vi "enigma.vi"() -> ()   [LabVIEW 2023]
panel:
  in  "Pistoketaulu":string[][](array[combo])
  in  "Kiekko 3":string(combo)
  in  "Kiekko 2":string(combo)
  in  "Kiekko 1":string(combo)
  in  "Kiekot":dbl[](array[numeric]) min=1.0 max=3.0 step=1.0
  in  "III":string(combo)
  in  "II":string(combo)
  in  "I":string(combo)
  out "Teksti ulos":string
  in  "Teksti sisään":string
  # "Aloitus"
  # "Kiekkojen asetukset"
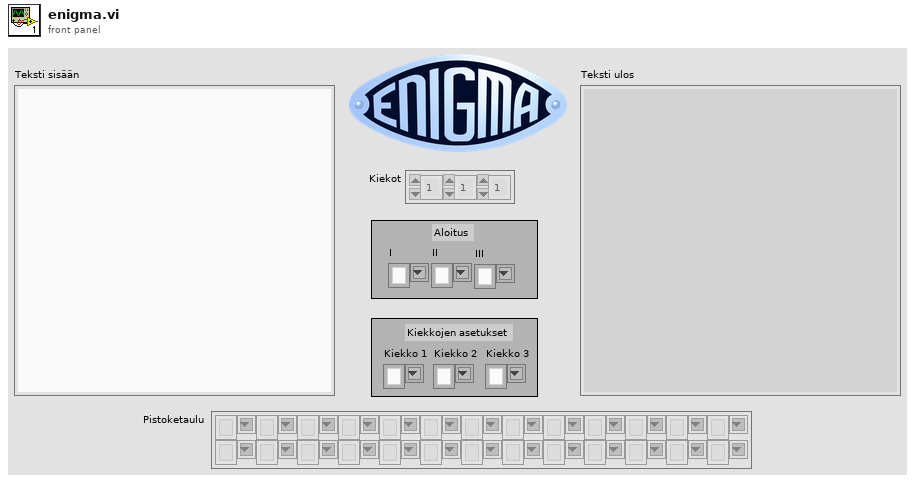
[diagram p1: front panel]
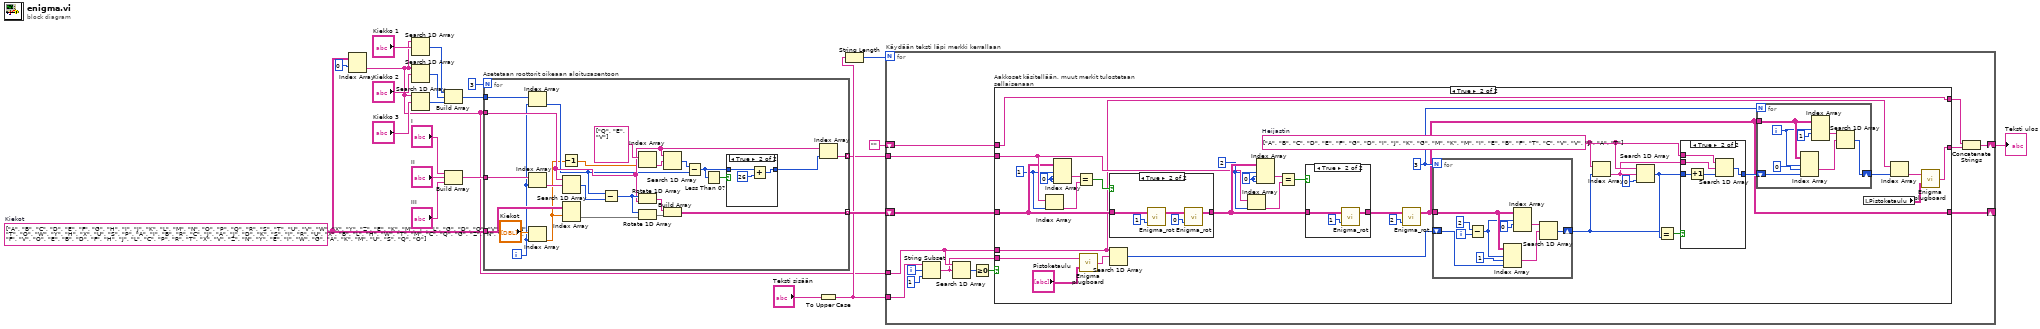
[diagram p0: block diagram]
diagram:
  w12 = string[][] [["A", "B", "C", "D", "E", "F", "G", "H", "I", "J", "K", "L", "M", "N", "O", "P", "Q", "R", "S", "T", "U", "V", "W", "X", "Y", "Z"], ["E", "K", "M", "F", "L", "G", "D", "Q", "V", "Z", "N", "T", "O", "W", "Y", "H", "X", "U", "S", "P", "A", "I", "B", "R", "C", "J"], ["A", "J", "D", "K", "S", "I", "R", "U", "X", "B", "L", "H", "W", "T", "M", "C", "Q", "G", "Z", "N", "P", "Y", "F", "V", "O", "E"], ["B", "D", "F", "H", "J", "L", "C", "P", "R", "T", "X", "V", "Z", "N", "Y", "E", "I", "W", "G", "A", "K", "M", "U", "S", "Q", "O"]]  # Kiekot
  n1 = Index Array(array=w12, index (row)=0) -> (element=w3:string[])  [unwired: 1 in]
  n2 = Search 1D Array(1D array=w3, element="Kiekko 1") -> (index of element=w7:i32)  [unwired: 1 in]
  n3 = Search 1D Array(1D array=w3, element="Kiekko 2") -> (index of element=w6:i32)  [unwired: 1 in]
  n4 = Search 1D Array(1D array=w3, element="Kiekko 3") -> (index of element=w5:i32)  [unwired: 1 in]
  n5 = Build Array(w7, w6, w5) -> (w4:i32[])
  n6 = Build Array("I", "II", "III") -> (w17:string[])
  n7 = for "Asetetaan roottorit oikeaan aloitusasentoon" {
    N: 3 -> [_]
    tunnel: w17 -> [w44]
    tunnel: [w40] -> w16 mode=indexing
    tunnel: w12 -> [w39]
    tunnel: w4 -> [w37]
    tunnel: w3 -> [w28]
    tunnel: [w34] -> w2 mode=indexing
    i -> [w23]
    n8 = Index Array(array=w37, index=w23) -> (element=w27:i32)
    n9 = Index Array(array=w44, index=w23) -> (element=w43:string)
    n10 = Index Array(array="Kiekot", index=w23) -> (element=w26:dbl)
    n11 = Decrement(x=w26) -> (x-1=w25:dbl)
    n12 = Search 1D Array(1D array=w28, element=w43) -> (index of element=w24:i32)  [unwired: 1 in]
    n13 = Index Array(array=w39, index (row)=w26) -> (element=w45:string[])  [unwired: 1 in]
    n14 = Subtract(x=w27, y=w24) -> (x-y=w33:i32)
    n15 = Index Array(array=string[] ["Q", "E", "V"], index=w25) -> (element=w35:string)
    n16 = Rotate 1D Array(1:w28, 2:w33) -> (0:w41:string[])
    n17 = Rotate 1D Array(1:w45, 2:w33) -> (0:w42:string[])
    n18 = Search 1D Array(1D array=w28, element=w35) -> (index of element=w32:i32)  [unwired: 1 in]
    n19 = Build Array(w41, w42) -> (w40:string[][])
    n20 = Subtract(x=w32, y=w27) -> (x-y=w30:i32)
    n21 = Less Than 0?(x=w30) -> (x < 0?=w31:bool)
    n22 = case shown="True" w31 {
      tunnel: w30 -> [w46 w49]
      tunnel: [w46 w47] -> w29
      frame False {
      }
      frame True {
        n23 = Add(x=w49, y=26) -> (x+y=w47:i32)
      }
    }
    n24 = Index Array(array=w28, index=w29) -> (element=w34:string)
  }
  n25 = To Upper Case(1:"Teksti sisään") -> (0:w13:string)
  n26 = String Length(string=w13) -> (length=w22:i32)
  n27 = for "Käydään teksti läpi merkki kerrallaan" {
    N: w22 -> [_]
    tunnel: w13 -> [w63]
    shift-right: [w53] -> w1
    shift-left: "" -> [w60]
    tunnel: w3 -> [w51]
    shift-right: [w58] -> _
    shift-left: w16 -> [w59]
    tunnel: w2 -> [w54]
    i -> [w62]
    n28 = String Subset(string=w63, offset (0)=w62, length (rest)=1 ("length (rest)")) -> (substring=w50:string)
    n29 = Search 1D Array(1D array=w51, element=w50) -> (index of element=w57:i32)  [unwired: 1 in]
    n30 = Greater Or Equal To 0?(x=w57) -> (x >= 0?=w56:bool)
    n31 = case "Aakkoset käsitellään, muut merkit tulostetaan sellaisenaan" shown="True" w56 {
      tunnel: w60 -> [w65 w93]
      tunnel: w51 -> [_ w67]
      tunnel: w59 -> [w66 w79]
      tunnel: [w66 w77] -> w58
      tunnel: [w65 w93] -> w55
      tunnel: [w64 w72] -> w52
      tunnel: w54 -> [_ w82]
      tunnel: w50 -> [w64 w69]
      frame False {
      }
      frame True {
        w80 = 0 ("disabled index (row)")
        w76 = 1 ("index")
        w84 = 0 ("disabled index (row)")
        w75 = 2 ("index (page)")
        w96 = string[] ["A", "B", "C", "D", "E", "F", "G", "D", "I", "J", "K", "G", "M", "K", "M", "I", "E", "B", "F", "T", "C", "V", "V", "J", "A", "T"]  # Heijastin
        w100 = 3
        n32 = Index Array(array=w82, index=w76) -> (element=w90:string)
        n33 = Index Array(array=w79, index (dim 0)=w76, index (dim 1)=w80, index (dim 2)=w80) -> (element=w81:string)
        n34 = Equal?(x=w81, y=w90) -> (x = y?=w89:bool)
        n35 = call "Enigma plugboard.vi"("Pistoketaulu"="Pistoketaulu", "Merkki sisään"=w69) -> ("Merkki ulos"=w68:string)
        n36 = case "Roottoreiden pyörittäminen" shown="True" w89 {
          tunnel: w79 -> [w105 w109]
          tunnel: [w105 w107] -> w85
          frame False {
          }
          frame True {
            n37 = call "Enigma_rot.vi"("Kiekon numero"=1 ("index (page)"), "Kiekot sisään"=w109) -> ("Kiekot ulos"=w108:string[][][])  [unwired: 1 in]
            n38 = call "Enigma_rot.vi"("Kiekon numero"=0 ("Roottorin numero"), "Kiekot sisään"=w108) -> ("Kiekot ulos"=w107:string[][][])  [unwired: 1 in]
          }
        }
        n39 = Search 1D Array(1D array=w67, element=w68) -> (index of element=w71:i32)  [unwired: 1 in]
        n40 = Index Array(array=w82, index=w75) -> (element=w87:string)
        n41 = Index Array(array=w85, index (dim 0)=w75, index (dim 1)=w84, index (dim 2)=w84) -> (element=w83:string)
        n42 = Equal?(x=w83, y=w87) -> (x = y?=w86:bool)
        n43 = case "Roottoreiden pyörittäminen" shown="True" w86 {
          tunnel: w85 -> [w101 w102]
          tunnel: [w101 w103] -> w78
          frame False {
          }
          frame True {
            n44 = call "Enigma_rot.vi"("Kiekon numero"=1 ("index (page)"), "Kiekot sisään"=w102) -> ("Kiekot ulos"=w103:string[][][])  [unwired: 1 in]
          }
        }
        n45 = call "Enigma_rot.vi"("Kiekon numero"=2 ("index (page)"), "Kiekot sisään"=w78) -> ("Kiekot ulos"=w77:string[][][])  [unwired: 1 in]
        n46 = for {
          N: w100 -> [_]
          tunnel: w77 -> [w131]
          shift-right: [w128] -> w88
          shift-left: w71 -> [w126]
          i -> [w130]
          n47 = Subtract(x=2, y=w130) -> (x-y=w129:i32)
          n48 = Index Array(array=w131, index (dim 0)=w129, index (dim 1)=1 ("disabled index (row)"), index (dim 2)=w126) -> (element=w125:string)
          n49 = Index Array(array=w131, index (dim 0)=w129, index (dim 1)=0 ("index (row)")) -> (element=w132:string[])  [unwired: 1 in]
          n50 = Search 1D Array(1D array=w132, element=w125) -> (index of element=w128:i32)  [unwired: 1 in]
        }
        n51 = Index Array(array=w96, index=w88) -> (element=w95:string)
        n52 = Search 1D Array(1D array=w96, element=w95, start index (0)=0) -> (index of element=w97:i32)
        n53 = Equal?(x=w88, y=w97) -> (x = y?=w98:bool)
        n54 = case shown="True" w98 {
          tunnel: w97 -> [w111 w115]
          tunnel: w96 -> [_ w114]
          tunnel: w95 -> [_ w113]
          tunnel: [w111 w112] -> w94
          frame False {
          }
          frame True {
            n55 = Increment(x=w115) -> (x+1=w116:i32)
            n56 = Search 1D Array(1D array=w114, element=w113, start index (0)=w116) -> (index of element=w112:i32)
          }
        }
        n57 = for {
          N: w100 -> [_]
          tunnel: w77 -> [w122]
          shift-right: [w119] -> w92
          shift-left: w94 -> [w120]
          i -> [w121]
          n58 = Index Array(array=w122, index (dim 0)=w121, index (dim 1)=0 ("disabled index (row)"), index (dim 2)=w120) -> (element=w118:string)
          n59 = Index Array(array=w122, index (dim 0)=w121, index (dim 1)=1 ("index (row)")) -> (element=w117:string[])  [unwired: 1 in]
          n60 = Search 1D Array(1D array=w117, element=w118) -> (index of element=w119:i32)  [unwired: 1 in]
        }
        n61 = local read "Pistoketaulu"() -> (w74:string[][])
        n62 = Index Array(array=w67, index=w92) -> (element=w73:string)
        n63 = call "Enigma plugboard.vi"("Pistoketaulu"=w74, "Merkki sisään"=w73) -> ("Merkki ulos"=w72:string)
      }
    }
    n64 = Concatenate Strings(w55, w52) -> (w53:string)
  }
  "Teksti ulos" <- w1
